vi "Example TDMS Read Events Data.vi"() -> ()   [LabVIEW 2019]
doc: "This example demonstrates how to read measured data, text and timestamps from a .tdms file using the TDMS API."
panel:
  out "Measured Data":waveform(dbl)[](graph)
  # "Overview: Demonstrates the use of the TDMS Read function to read measured data, text and timestamps from an existing .tdms file.\nInstructions:\n1. Make sure you have already run TDMS Write Events Data.vi.\n2. Run this VI.\n3. Delete the .tdms file (located at [LabVIEW Data]\\Example Events Data.tdms) when you are done."
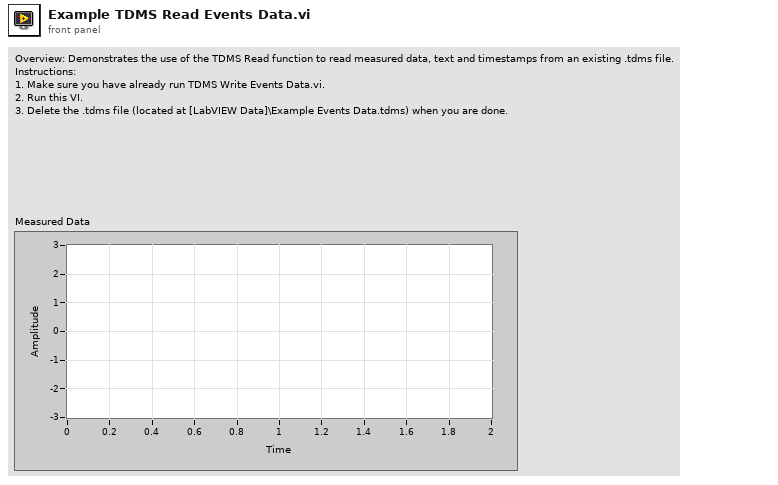
[diagram p1: front panel]
types:
  T1 = enum16{"open", "open or create", "create or replace", "create", "open (read-only)"}
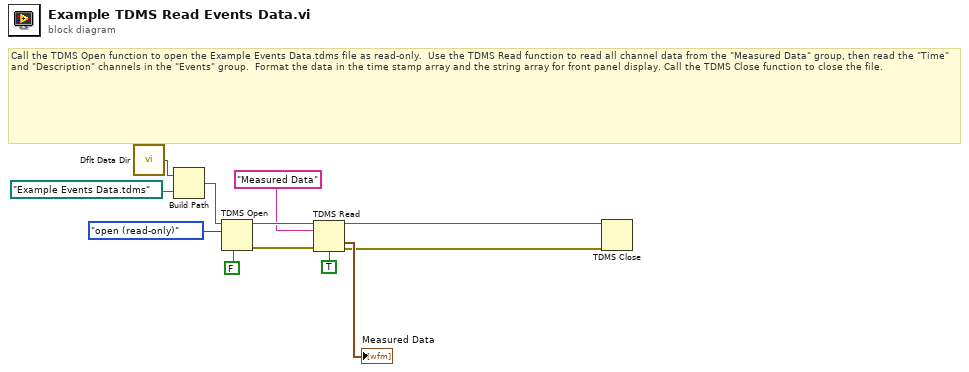
[diagram p0: block diagram]
diagram:
  # "Call the TDMS Open function to open the Example Events Data.tdms file as read-only.  Use the TDMS Read function to read all channel data from the \"Measured Data\" group, then read the \"Time\" and \"Description\" channels in the \"Events\" group.  Format the data in the time stamp array and the string array for front panel display. Call the TDMS Close function to close the file."
  n1 = call <vilib>:"Dflt Data Dir.vi"() -> ("App:Default Data Directory"=w12:path)
  n2 = Build Path(base path=w12, name or relative path=path "Example Events Data.tdms" ("file path")) -> (appended path=w6:path)
  n3 = TDMS Open(6:FALSE ("disable buffering (T)"), 10:T1."open (read-only)" ("operation"), 11:w6) -> (0:w8:errorcluster, 3:w9:refnum<k34>)  [unwired: 4 in]
  n4 = TDMS Read(0:w9, 5:"Measured Data" ("group name"), 11:w8, 13:TRUE ("return channels in file order? (F)")) -> (4:w2:refnum<k34>, 10:→"Measured Data":waveform(dbl)[], 15:w1:errorcluster)  [unwired: 4 in, 3 out]
  n5 = TDMS Close(8:w1, 11:w2) -> ()  [unwired: 2 out]
